vi "find_circles.vi"(5 "shrinkFactor":i32, 6 "Field of View":cluster{"fieldOfViewX":sgl, "fieldOfViewY":sgl}, 7 "logFileDir":string, 8 "error in":errorcluster, 9 "debug":bool, 10 "find_circles parameters":T2, 11 "Image":T3) -> (0 "error out":errorcluster, 2 "Circles":T1(array[cluster]))   [LabVIEW 2017, in "gVision.lvlib"]
uses:
  gVision.lvlib
  <vilib>/vision/Image Controls.llb/IMAQ Image.ctl
  find_circles parameters.ctl
panel:
  # "Image must be an 8-bin greyscale image"
  # "For error circle"
  # "in micrometers"
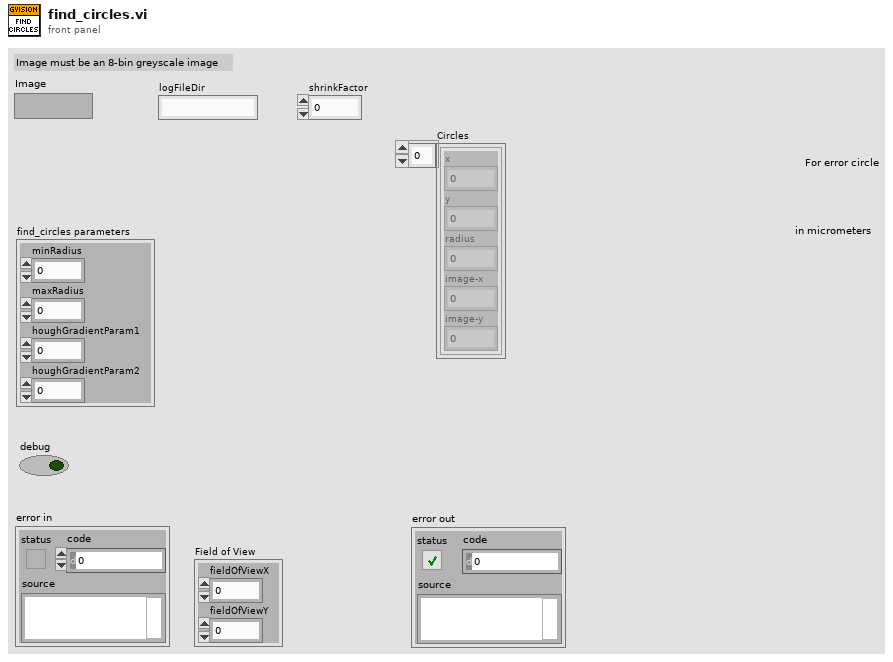
[diagram p1: front panel]
types:
  T1 = cluster{"x":dbl, "y":dbl, "radius":dbl, "image-x":dbl, "image-y":dbl}[]
  T2 = typedef "find_circles parameters.ctl" = cluster{"minRadius":sgl, "maxRadius":sgl, "houghGradientParam1":i32, "houghGradientParam2":i32}
  T3 = typedef "IMAQ Image.ctl" = refnum<image>
  T4 = enum32{"Map Pixel Pointer", "Unmap Pixel Pointer", "Get Pixels Infos"}
  T5 = cluster{"x":dbl, "y":dbl, "radius":dbl, "image-x":dbl, "image-y":dbl}
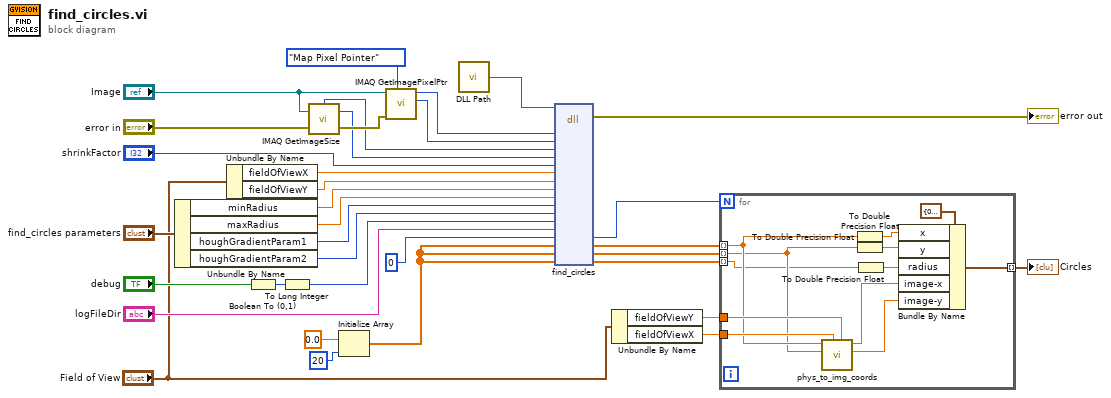
[diagram p0: block diagram]
diagram:
  n1 = Unbundle By Name("find_circles parameters") -> ("minRadius"=w22:sgl, "maxRadius"=w21:sgl, "houghGradientParam1"=w20:i32, "houghGradientParam2"=w19:i32)
  n2 = Unbundle By Name("Field of View") -> ("fieldOfViewX"=w2:sgl, "fieldOfViewY"=w1:sgl)
  n3 = Boolean To (0,1)(Boolean="debug") -> (0, 1=w23:i16)
  n4 = To Long Integer(number=w23) -> (32bit integer=w18:i32)
  n5 = call "IMAQ GetImageSize"("Image"="Image", "error in (no error)"="error in") -> ("Y Resolution"=w29:i32, "X Resolution"=w28:i32, "error out"=w30:errorcluster)  [unwired: 2 in]
  n6 = Initialize Array(sgl 0.0 ("element"), 20 ("dimension size")) -> (w14:sgl[])
  n7 = call "IMAQ GetImagePixelPtr"("Function"=T4."Map Pixel Pointer", "error in (no error)"=w30, "Image"="Image") -> ("LineWidth(Pixels)"=w27:i32, "Pixel Pointer out"=w26:u64)  [unwired: 3 in, 4 out]
  n8 = call "DLL Path.vi"() -> ("DLL Path"=w34:path)  [unwired: 5 in]
  n9 = dll-call lib="?" fn="find_circles"(path in=w34, "img"=w26, "imgLineWidth"=w27, "imgWidth"=w28, "imgHeight"=w29, "shrinkFactor"="shrinkFactor", "fieldOfViewX"=w2, "fieldOfViewY"=w1, "minRadius"=w22, "maxRadius"=w21, "houghGradientParam1"=w20, "houghGradientParam2"=w19, "debug"=w18, "logFileDir"="logFileDir", "numCircles"=0, "circleXCenters"=w14, "circleYCenters"=w14, "circleRadii"=w14) -> (error out=→"error out":errorcluster, "numCircles"=w9:i32, "circleXCenters"=w8:sgl[], "circleYCenters"=w7:sgl[], "circleRadii"=w6:sgl[])  [unwired: 16 in, 1 out]
  n10 = Unbundle By Name("Field of View") -> ("fieldOfViewY"=w12:sgl, "fieldOfViewX"=w11:sgl)
  n11 = for {
    N: w9 -> [_]
    tunnel: w8 -> [w39] mode=indexing
    tunnel: w7 -> [w36] mode=indexing
    tunnel: [w46] -> w5 mode=indexing
    tunnel: w12 -> [w41]
    tunnel: w11 -> [w40]
    tunnel: w6 -> [w35] mode=indexing
    n12 = call "phys_to_img_coords.vi"("fov_y"=w41, "fov_x"=w40, "y"=w36, "x"=w39) -> ("image_y"=w37:dbl, "image_x"=w38:dbl)  [unwired: 6 in]
    n13 = To Double Precision Float(number=w39) -> (double precision float=w45:dbl)
    n14 = To Double Precision Float(number=w36) -> (double precision float=w44:dbl)
    n15 = To Double Precision Float(number=w35) -> (double precision float=w43:dbl)
    n16 = Bundle By Name(cluster=T5 {"x"=0.0, "y"=0.0, "radius"=0.0, "image-x"=0.0, "image-y"=0.0}, "x"=w45, "y"=w44, "radius"=w43, "image-x"=w38, "image-y"=w37) -> (w46:T5)
  }
  "Circles" <- w5
